vi "ex04_ITEM.vi"() -> ()   [LabVIEW 2011]
panel:
  out "Numeric 6":dbl
  out "Numeric 5":dbl
  in  "Numeric 4":dbl
  in  "Numeric 3":dbl
  in  "Numeric 2":dbl
  in  "Numeric":dbl
  in  "stop":bool
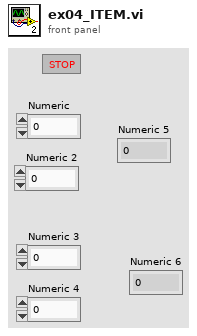
[diagram p1: front panel]
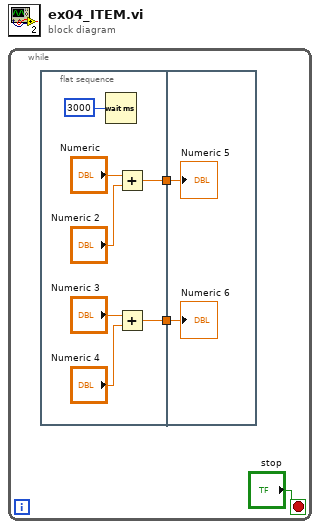
[diagram p0: block diagram]
diagram:
  n1 = while {
    stop <- "stop" stop-if-true
    n2 = flat-sequence {
      tunnel: [w6] -> w2
      tunnel: [w5] -> w1
      tunnel: w2 -> [w12]
      tunnel: w1 -> [w11]
      frame #0 {
        n3 = Wait (ms)(milliseconds to wait=u32 3000) -> ()  [unwired: 1 out]
        n4 = Add(x="Numeric", y="Numeric 2") -> (x+y=w6:dbl)
        n5 = Add(x="Numeric 3", y="Numeric 4") -> (x+y=w5:dbl)
      }
      frame #1 {
        "Numeric 5" <- w12
        "Numeric 6" <- w11
      }
    }
  }
